vi "Configuration Write.vi"(7 "Digit Resolution(5½)":T1=enum."5½", 8 "error in (no error)":errorcluster, 9 "Range":dbl, 10 "Function":T2, 11 "DMM Driver in":refnum<class "DMM Driver.lvclass">) -> (0 "error out":errorcluster, 1 "Success?":bool, 3 "DMM Driver out":refnum<class "DMM Driver.lvclass">)   [LabVIEW 2020, in "DMM.lvlib" / "DMM Driver.lvclass"]
doc: "Check if the configuration should be changed and if the change is allowed. If both checks are OK the configuration is changed using 'Configuration Write Do'."
uses:
  DMM Driver.lvclass
  Controls/Ctl_Function.ctl
  DMM.lvlib
  Controls/Ctl_DigitResolution.ctl
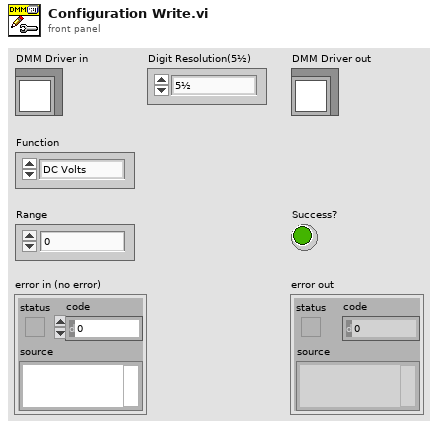
[diagram p1: front panel]
types:
  T1 = typedef "DMM.lvlib/Ctl_DigitResolution.ctl" = enum8{"3½", "4½", "5½", "6½", "7½"}
  T2 = typedef "DMM.lvlib/Ctl_Function.ctl" = enum8{"DC Volts", "AC Volts", "DC Current", "AC Current", "2-wire Resistance", "4-wire Resistance", "Diode", "Frequency", "Period", "AC Volts DC Coupled", "Capacitance", "Inductance", "Temperature"}
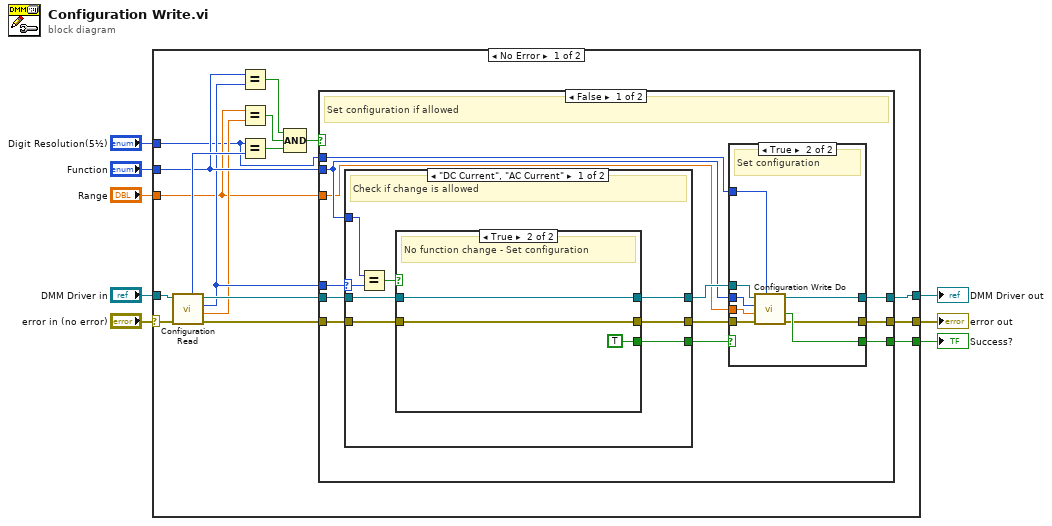
[diagram p0: block diagram]
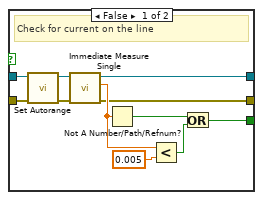
[diagram p3: hidden frame]
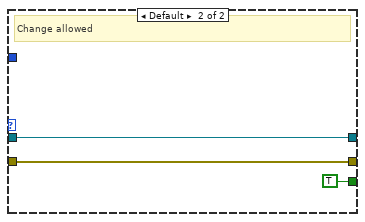
[diagram p4: hidden frame]
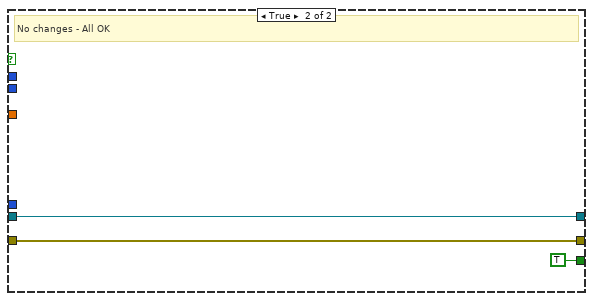
[diagram p5: hidden frame]
diagram:
  n1 = case shown="No Error" "error in (no error)" {
    selector: "error in (no error)" -> [w18 w78]
    tunnel: "DMM Driver in" -> [w25 w77]
    tunnel: [w24 w77] -> w7
    tunnel: "Function" -> [w21 _]
    tunnel: [w13 _] -> w4
    tunnel: [w12 w78] -> w3
    tunnel: "Range" -> [w10 _]
    tunnel: "Digit Resolution(5½)" -> [w9 _]
    frame No Error {
      n2 = call-dynamic "Configuration Read.vi"("error in (no error)"=w18, "DMM Driver in"=w25) -> ("error out"=w11:errorcluster, "Range"=w19:dbl, "Function"=w20:T2, "DMM Driver out"=w23:refnum<class "DMM Driver.lvclass">, "Digit Resolution(5½)"=w22:T1)  [unwired: 5 in]
      n3 = Equal?(x=w21, y=w20) -> (x = y?=w17:bool)
      n4 = Equal?(x=w10, y=w19) -> (x = y?=w16:bool)
      n5 = Equal?(x=w9, y=w22) -> (x = y?=w15:bool)
      n6 = Compound Arithmetic op=AND(w17, w16, w15) -> (w14:bool)
      n7 = case shown="False" w14 {
        tunnel: [w32 w76] -> w24
        tunnel: w23 -> [w37 w76]
        tunnel: w21 -> [w28 _]
        tunnel: w20 -> [w36 _]
        tunnel: [w33 TRUE ("Success?")] -> w13
        tunnel: [w30 w74] -> w12
        tunnel: w11 -> [w35 w74]
        tunnel: w10 -> [w27 _]
        tunnel: w9 -> [w26 _]
        frame False {
          # "Set configuration if allowed"
          n8 = case shown="\"DC Current\", \"AC Current\"" w36 {
            selector: w36 -> [w55 _]
            tunnel: w28 -> [w56 _]
            tunnel: [w50 w73] -> w31
            tunnel: w37 -> [w53 w73]
            tunnel: [w49 w72] -> w29
            tunnel: w35 -> [w52 w72]
            tunnel: [w51 TRUE] -> w34
            frame "DC Current", "AC Current" {
              # "Check if change is allowed"
              n9 = Equal?(x=w56, y=w55) -> (x = y?=w54:bool)
              n10 = case shown="True" w54 {
                tunnel: w53 -> [w67 w69]
                tunnel: w52 -> [w65 w68]
                tunnel: [w59 TRUE] -> w51
                tunnel: [w58 w69] -> w50
                tunnel: [w57 w68] -> w49
                frame False {
                  # "Check for current on the line"
                  n11 = call-dynamic "Set Autorange.vi"("error in (no error)"=w65, "DMM Driver in"=w67) -> ("error out"=w64:errorcluster, "DMM Driver out"=w66:refnum<class "DMM Driver.lvclass">)  [unwired: 8 in]
                  n12 = call-dynamic "Immediate Measure Single.vi"("error in (no error)"=w64, "DMM Driver in"=w66) -> ("error out"=w57:errorcluster, "Measurement"=w62:dbl, "DMM Driver out"=w58:refnum<class "DMM Driver.lvclass">)  [unwired: 5 in, 2 out]
                  n13 = Not A Number/Path/Refnum?(number/path/refnum=w62) -> (NaN/Path/Refnum?=w60:bool)
                  n14 = Less?(x=w62, y=0.005) -> (x < y?=w61:bool)
                  n15 = Or(x=w60, y=w61) -> (x .or. y?=w59:bool)
                }
                frame True {
                  # "No function change - Set configuration"
                }
              }
            }
            frame Default {
              # "Change allowed"
            }
          }
          n16 = case shown="True" w34 {
            selector: w34 -> [w40 _]
            tunnel: [w40 w46] -> w33
            tunnel: [w39 w47] -> w32
            tunnel: w31 -> [w39 w48]
            tunnel: [w38 w44] -> w30
            tunnel: w29 -> [w38 w45]
            tunnel: w28 -> [_ w43]
            tunnel: w27 -> [_ w42]
            tunnel: w26 -> [_ w41]
            frame False {
              # "Change not allowed"
            }
            frame True {
              # "Set configuration"
              n17 = call-dynamic "Configuration Write Do.vi"("Digit Resolution(5½)"=w41, "error in (no error)"=w45, "Range"=w42, "Function"=w43, "DMM Driver in"=w48) -> ("error out"=w44:errorcluster, "Success?"=w46:bool, "DMM Driver out"=w47:refnum<class "DMM Driver.lvclass">)  [unwired: 4 in]
            }
          }
        }
        frame True {
          # "No changes - All OK"
        }
      }
    }
    frame Error {
    }
  }
  "error out" <- w3
  "DMM Driver out" <- w7
  "Success?" <- w4
